vi "Check_Lengths_of_Subtracks-1.vi"(1 "[IN] Subtracks":T1(array[cluster]), 2 "[IN] Number of Additi\nonal Costs (Subtracks)":i32) -> (0 "[OUT[ Is between subtracks\npresented too short one?":bool)   [LabVIEW 2013]
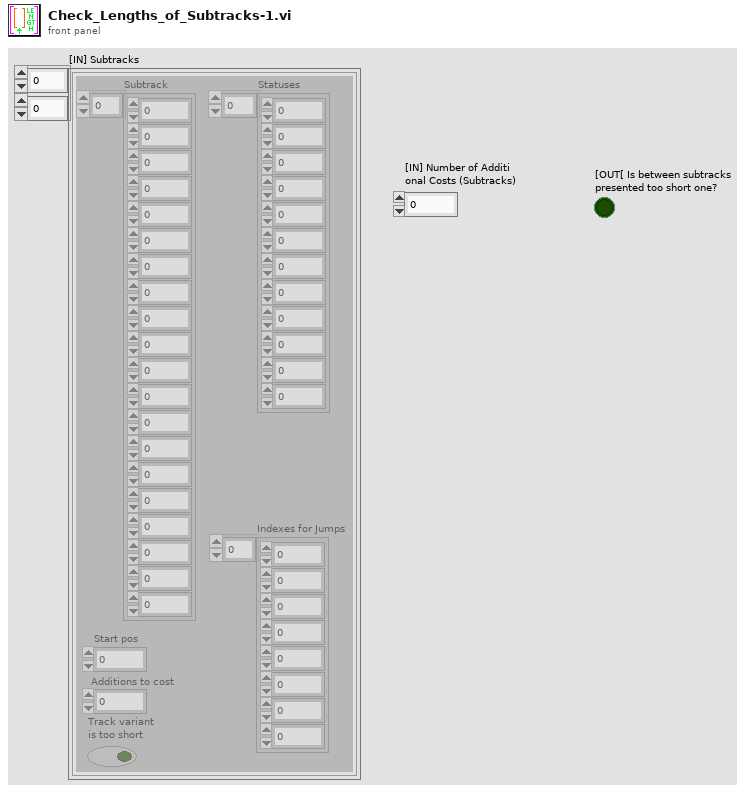
[diagram p1: front panel]
types:
  T1 = cluster{"Subtrack":dbl[], "Statuses":i16[], "Start pos":i32, "Additions to cost":i32, "Track variant \nis too short":bool, "Indexes for Jumps":i32[]}[][]
  T2 = cluster{"Subtrack":dbl[], "Statuses":i16[], "Start pos":i32, "Additions to cost":i32, "Track variant \nis too short":bool, "Indexes for Jumps":i32[]}[]
  T3 = cluster{"Subtrack":dbl[], "Statuses":i16[], "Start pos":i32, "Additions to cost":i32, "Track variant \nis too short":bool, "Indexes for Jumps":i32[]}
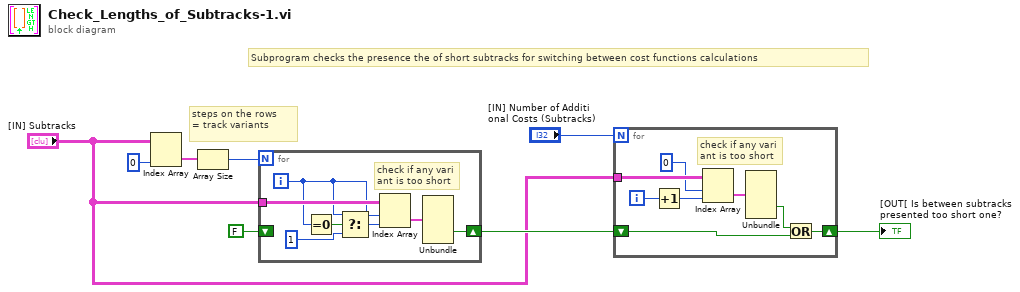
[diagram p0: block diagram]
diagram:
  # "Subprogram checks the presence the of short subtracks for switching between cost functions calculations"
  # "steps on the rows\n= track variants"
  n1 = Index Array(array="[IN] Subtracks", index (col)=0 ("disabled index (col)")) -> (element=w7:T2)  [unwired: 1 in]
  n2 = Array Size(array=w7) -> (size(s)=w5:i32)
  n3 = for {
    N: w5 -> [_]
    tunnel: "[IN] Subtracks" -> [w15]
    shift-right: [w13] -> w4
    shift-left: FALSE -> [_]
    i -> [w9]
    # "check if any vari\nant is too short"
    n4 = Equal To 0?(x=w9) -> (x = 0?=w12:bool)
    n5 = Select(t=w9, s=w12, f=1) -> (s? t:f=w10:i32)
    n6 = Index Array(array=w15, index (row)=w9, index (col)=w10) -> (element=w14:T3)
    n7 = Unbundle(w14) -> ("Track variant \nis too short"=w13:bool)  [unwired: 5 out]
  }
  n8 = for {
    N: "[IN] Number of Additi\nonal Costs (Subtracks)" -> [_]
    tunnel: "[IN] Subtracks" -> [w23]
    shift-right: [w19] -> w1
    shift-left: w4 -> [w20]
    i -> [w17]
    # "check if any vari\nant is too short"
    n9 = Increment(x=w17) -> (x+1=w16:i32)
    n10 = Index Array(array=w23, index (row)=0 ("disabled index (row)"), index (col)=w16) -> (element=w22:T3)
    n11 = Unbundle(w22) -> ("Track variant \nis too short"=w18:bool)  [unwired: 5 out]
    n12 = Or(x=w18, y=w20) -> (x .or. y?=w19:bool)
  }
  "[OUT[ Is between subtracks\npresented too short one?" <- w1
